vi "Open Connection_SALTOPIC.vi"(8 "error in (no error)":errorcluster, 9 "SALTOPIC":T1, 10 "topicName":string) -> (0 "error out":errorcluster, 3 "topicRef":cluster{"topicName":string, "type":refnum<vi>})   [LabVIEW 2015]
uses:
  SALTypedefs/SALDATA/SALTOPIC.ctl
  SALTypedefs/SALDATA/SALDATA.lvlib
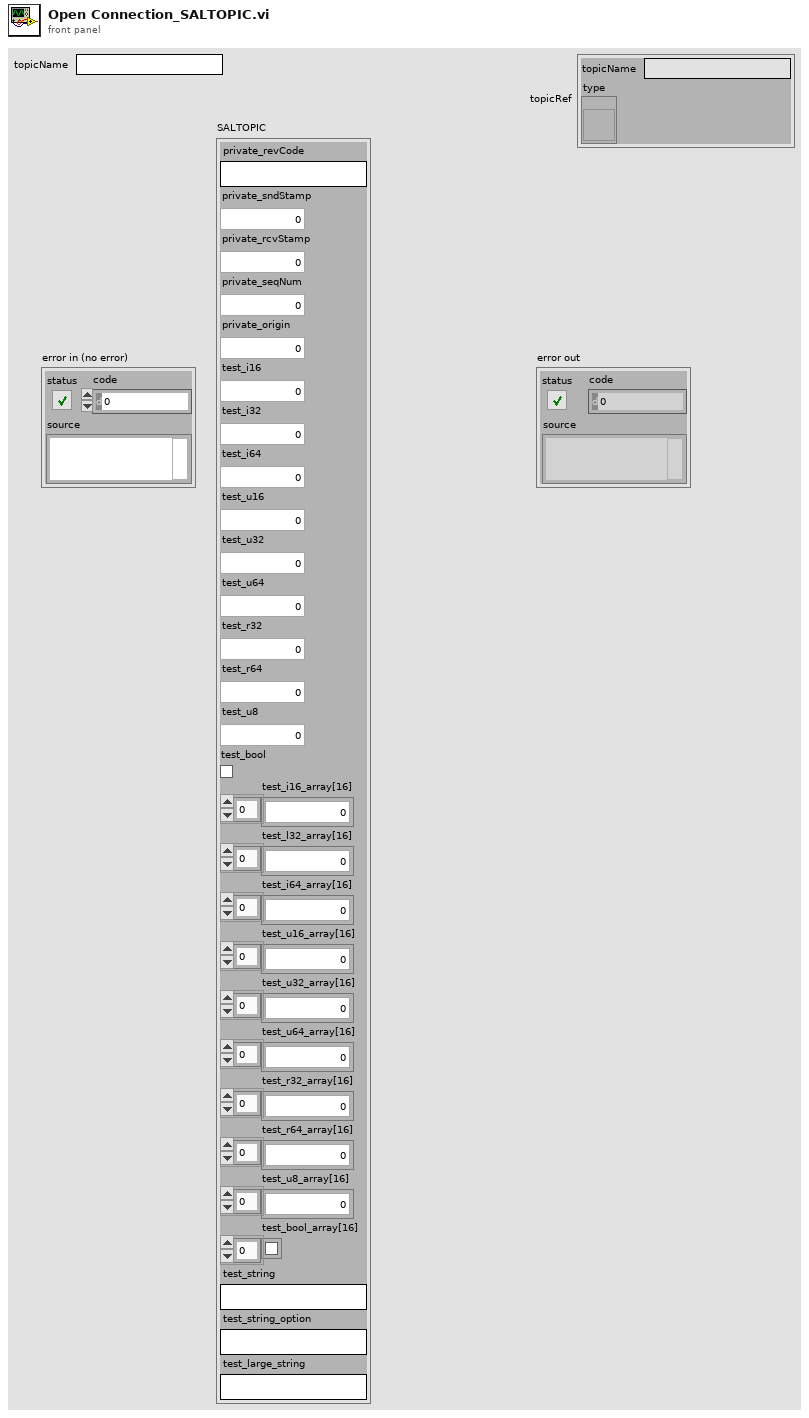
[diagram p1: front panel]
types:
  T1 = typedef "SALDATA.lvlib/SALTOPIC.ctl" = cluster{"private_revCode":string, "private_sndStamp":dbl, "private_rcvStamp":dbl, "private_seqNum":i32, "private_origin":i32, "test_i16":i16, "test_i32":i32, "test_i64":i64, "test_u16":u16, "test_u32":u32, "test_u64":u64, "test_r32":sgl, "test_r64":dbl, "test_u8":u8, "test_bool":bool, "test_i16_array[16]":i16[], "test_l32_array[16]":i32[], "test_i64_array[16]":i64[], "test_u16_array[16]":u16[], "test_u32_array[16]":u32[], "test_u64_array[16]":u64[], "test_r32_array[16]":sgl[], "test_r64_array[16]":dbl[], "test_u8_array[16]":u8[], "test_bool_array[16]":bool[], "test_string":string, "test_string_option":string, "test_large_string":string}
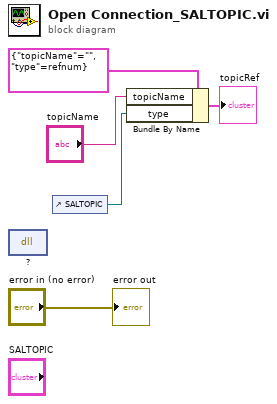
[diagram p0: block diagram]
diagram:
  n1 = dll-call lib="?" fn="?"() -> ()  [unwired: 4 in, 2 out]
  n2 = control-ref of="SALTOPIC"() -> (w2:refnum<vi>)
  n3 = Bundle By Name(cluster=cluster{"topicName":string, "type":refnum<vi>} {"topicName"="", "type"=refnum} ("topicRef"), "topicName"="topicName", "type"=w2) -> (→"topicRef":cluster{"topicName":string, "type":refnum<vi>})
  "error out" <- "error in (no error)"
